vi "Format and Append Version String.vi"(6 "Version":T1 {"Build Date/Time" format="%<%X\n%x>T"}, 9 "String (Empty)":string) -> (0 "String with Version & Build":string, 1 "String with Version":string)   [LabVIEW 2011]
uses:
  OGAB Version.ctl
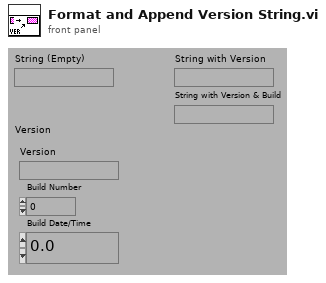
[diagram p1: front panel]
types:
  T1 = typedef "OGAB Version.ctl" = cluster{"Version":string, "Build Number":u32, "Build Date/Time":dbl}
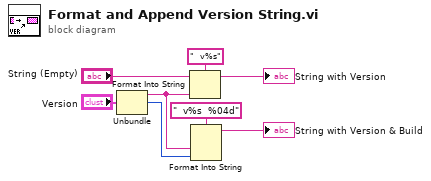
[diagram p0: block diagram]
diagram:
  n1 = Unbundle("Version") -> ("Version"=w4:string, "Build Number"=w3:u32)  [unwired: 1 out]
  n2 = Format Into String(format string="  v%s", initial string="String (Empty)", w4) -> (resulting string=→"String with Version":string)  [unwired: 1 in, 1 out]
  n3 = Format Into String(format string="  v%s  %04d", w4, w3) -> (resulting string=→"String with Version & Build":string)  [unwired: 2 in, 1 out]
